vi "GPIB_Read.vi"(0 "address string":string, 1 "byte count":i32, 2 "mode (0)":i16, 3 "error in":errorcluster, 4 "timeout ms (488.2 global)":i32=2000) -> (5 "data Out":string, 6 "status":bool[](array[boolean]), 7 "error out":errorcluster)   [LabVIEW 2011]
uses:
  Controls/GPIB_Mode.ctl
  Globals/Dynamic_call_global.ph.vi
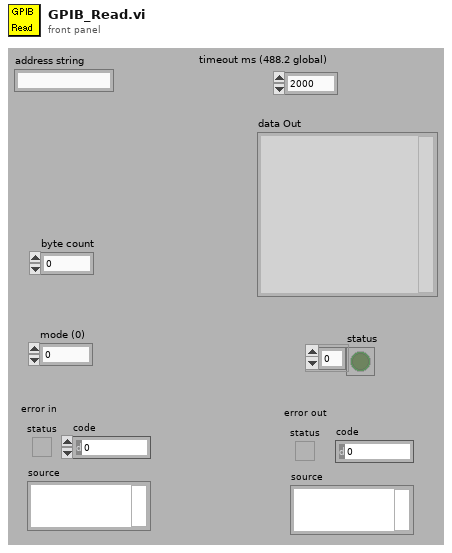
[diagram p1: front panel]
types:
  T1 = typedef "GPIB_Mode.ctl" = enum16{"Read", "Write", "Trigger", "Poll"}
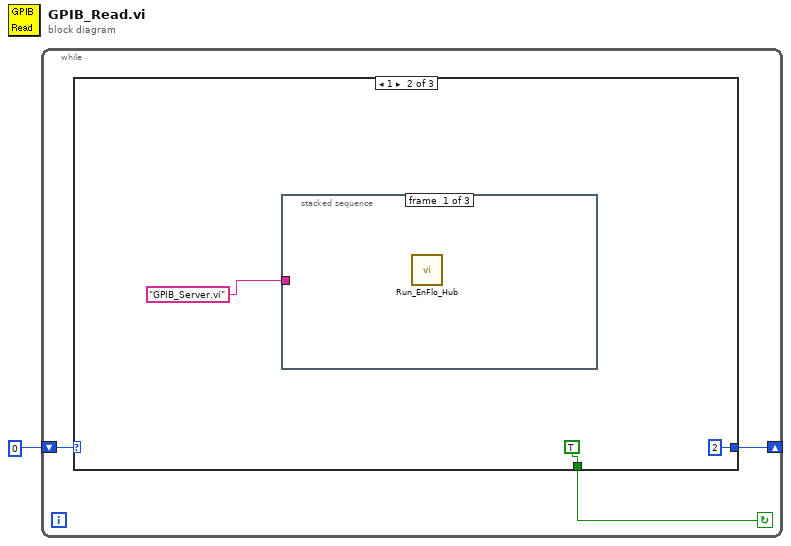
[diagram p0: block diagram]
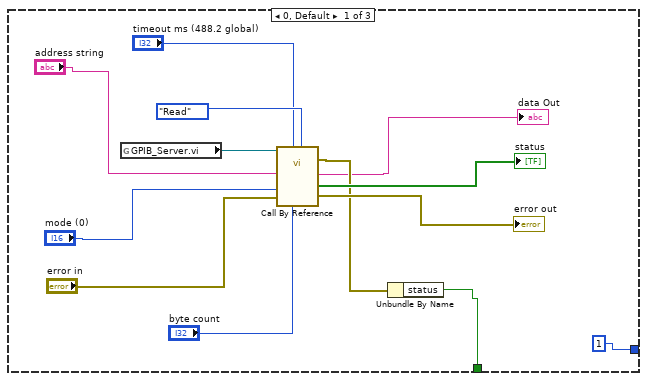
[diagram p2: hidden frame]
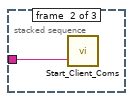
[diagram p3: hidden frame]
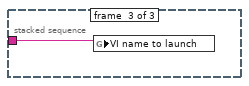
[diagram p4: hidden frame]
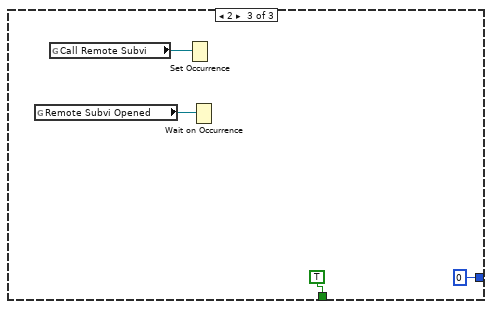
[diagram p5: hidden frame]
diagram:
  n1 = while {
    shift-right: [w3] -> _
    shift-left: 0 -> [w4]
    stop <- w2 continue-if-true
    n2 = case shown="1" w4 {
      tunnel: [1 2 0] -> w3
      tunnel: [w7 TRUE ("status") TRUE ("status")] -> w2
      frame 0, Default {
        n3 = global read "Dynamic_call_global.ph.vi" "GPIB_Server.vi"() -> (w17:refnum<vi>)
        n4 = call-by-ref "?"(reference=w17, "Case"=GPIB_Mode."Read", "byte count"="byte count", "error in"="error in", "mode (0)"="mode (0)", "timeout ms (488.2 global)"="timeout ms (488.2 global)", "address string"="address string") -> (error out=w9:errorcluster, 0:"error out"=→"error out":errorcluster, "status"=→"status":bool[], "data Out"=→"data Out":string)  [unwired: 3 in, 1 out]
        n5 = Unbundle By Name(w9) -> ("status"=w7:bool)
      }
      frame 1 {
        n6 = stacked-sequence {
          tunnel: "GPIB_Server.vi" ("VI name to launch") -> [_ w21 w22]
          frame #0 {
            n7 = call "Run_EnFlo_Hub.vi"() -> ()  [unwired: 8 out]
          }
          frame #1 {
            n8 = call "Start_Client_Coms.vi"("VI name to run on server"=w21) -> ()  [unwired: 1 in, 4 out]
          }
          frame #2 {
            n9 = global write "Dynamic_call_global.ph.vi" "VI name to launch"(w22) -> ()
          }
        }
      }
      frame 2 {
        n10 = global read "Dynamic_call_global.ph.vi" "Remote Subvi Opened"() -> (w25:refnum<k4>)
        n11 = global read "Dynamic_call_global.ph.vi" "Call Remote Subvi"() -> (w26:refnum<k4>)
        n12 = Set Occurrence(w26) -> ()
        n13 = Wait on Occurrence(2:w25) -> ()  [unwired: 3 out]
      }
    }
  }
